vi "tutorial 5.vi"() -> ()   [LabVIEW 2022 SP3]
panel:
  out "Output":string
  in  "User Input":string
  in  "function name":string
  in  "Python version":string
  # "slicing 0:4"
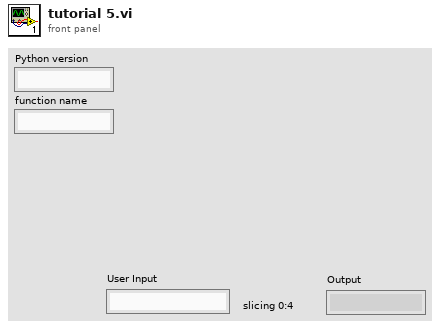
[diagram p1: front panel]
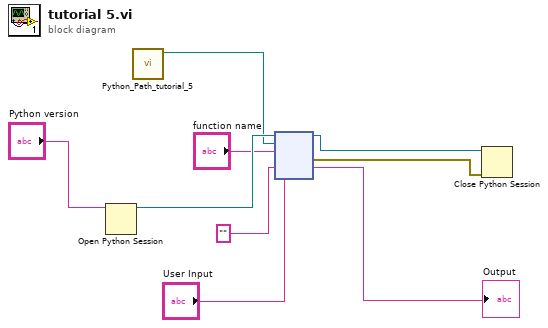
[diagram p0: block diagram]
diagram:
  n1 = Open Python Session(python version="Python version") -> (session out=w8:refnum<k35>)  [unwired: 2 in, 1 out]
  n2 = call "Python_Path_tutorial_5.vi"() -> ("appended path"=w6:path)  [unwired: 11 in]
  n3 = node(w8, w6, "function name", "", "User Input") -> (w7:refnum<k35>, w4:errorcluster, →"Output":string)  [unwired: 2 in, 2 out]
  n4 = Close Python Session(session in=w7, error in=w4) -> ()  [unwired: 1 out]
